vi "armstrong number.vi"() -> ()   [LabVIEW 2020]
panel:
  out "sum":dbl
  in  "Numeric":dbl
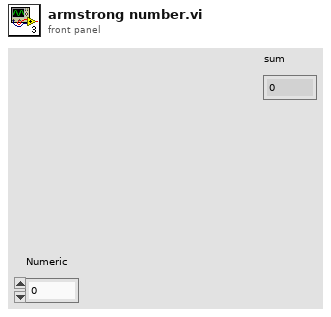
[diagram p1: front panel]
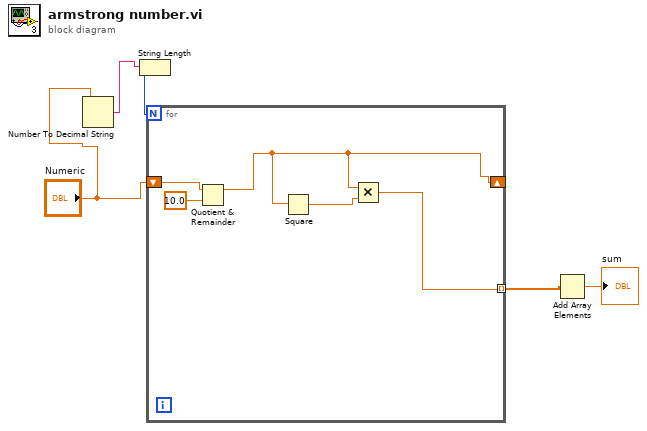
[diagram p0: block diagram]
diagram:
  n1 = Number To Decimal String(number="Numeric") -> (decimal integer string=w2:string)  [unwired: 1 in]
  n2 = String Length(string=w2) -> (length=w1:i32)
  n3 = for {
    N: w1 -> [_]
    shift-right: [w6] -> _
    shift-left: "Numeric" -> [w9]
    tunnel: [w7] -> w5 mode=indexing
    n4 = Quotient & Remainder(x=w9, y=10.0) -> (x-y*floor(x/y)=w6:dbl)  [unwired: 1 out]
    n5 = Square(x=w6) -> (x^2=w8:dbl)
    n6 = Multiply(x=w6, y=w8) -> (x*y=w7:dbl)
  }
  n7 = Add Array Elements(numeric array=w5) -> (sum=→"sum":dbl)
